vi "Get Goal Positions.vi"(11 "Game Board in":refnum<class "Game Board.lvclass">) -> (1 "Width goal out":u16, 2 "Bounds out":T1)   [LabVIEW 2024, in "Game Board.lvclass"]
doc: "MIT Licence\nCopyright (c) 2024 David Grollier"
uses:
  Game Board.lvclass
  <vilib>/Utility/miscctls.llb/LVBoundsTypeDef.ctl
  Game Board.lvclass/Game Board.ctl
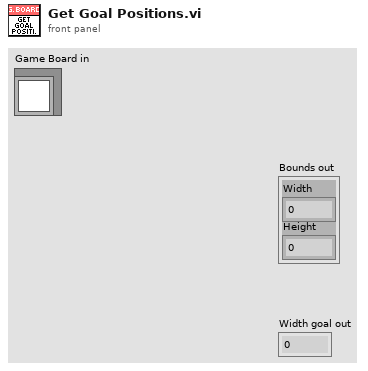
[diagram p1: front panel]
types:
  T1 = typedef "LVBoundsTypeDef.ctl" = cluster{"Width":u32, "Height":u32}
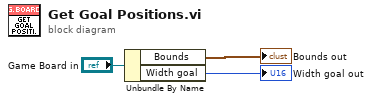
[diagram p0: block diagram]
diagram:
  n1 = Unbundle By Name("Game Board in") -> ("Bounds"=→"Bounds out":T1, "Width goal"=→"Width goal out":u16)
